vi "Data2Arrays.vi"(8 "error in (no error)":errorcluster, 11 "AllData":T1 {"FlukeData"."DataAnalysisArray"."TimeStamp" format="%^<%.3X\n%x>T"; "FlukeData"."ModelDataArray"."FREQUENCY" format="%#_6f"; "FlukeData"."ModelDataArray"."TimeStamp" format="%^<%.3X\n%x>T"; "FlukeData"."PMUDataArray"."FREQUENCY" format="%#_6f"; "FlukeData"."PMUDataArray"."TimeStamp" format="%^<%.3X\n%x>T"; "NISTData"."DataAnlysisArray"."Time" format="%.6f"; "NISTData"."DataAnlysisArray"."TimeStamp" format="%^<%.3X\n%x>T"; "NISTData"."DUTDataArray"."TimeStamp" format="%^<%.3X\n%x>T"; "NISTData"."DUTDataArray"."Time" format="%.6f"; "NISTData"."NIDataArray"."TimeStamp" format="%^<%.3X\n%x>T"; "NISTData"."NIDataArray"."Time" format="%.6f"}) -> (0 "error out":errorcluster, 2 "Fluke":dbl[][](array[numeric]), 3 "NIST":dbl[][](array[numeric]))   [LabVIEW 2014]
uses:
  typedefs/Alldata.ctl
  typedefs/NISTData.ctl
  typedefs/NIDataArray.ctl
  typedefs/NIData.ctl
  typedefs/PhasorRectangular.ctl
  typedefs/DUTData.ctl
  typedefs/NICalcAnalysis.ctl
  typedefs/CalcPhasorError.ctl
  typedefs/PlotDataArrays.ctl
  typedefs/PmuRawDataCluster.ctl
  typedefs/CalcAnalysis.ctl
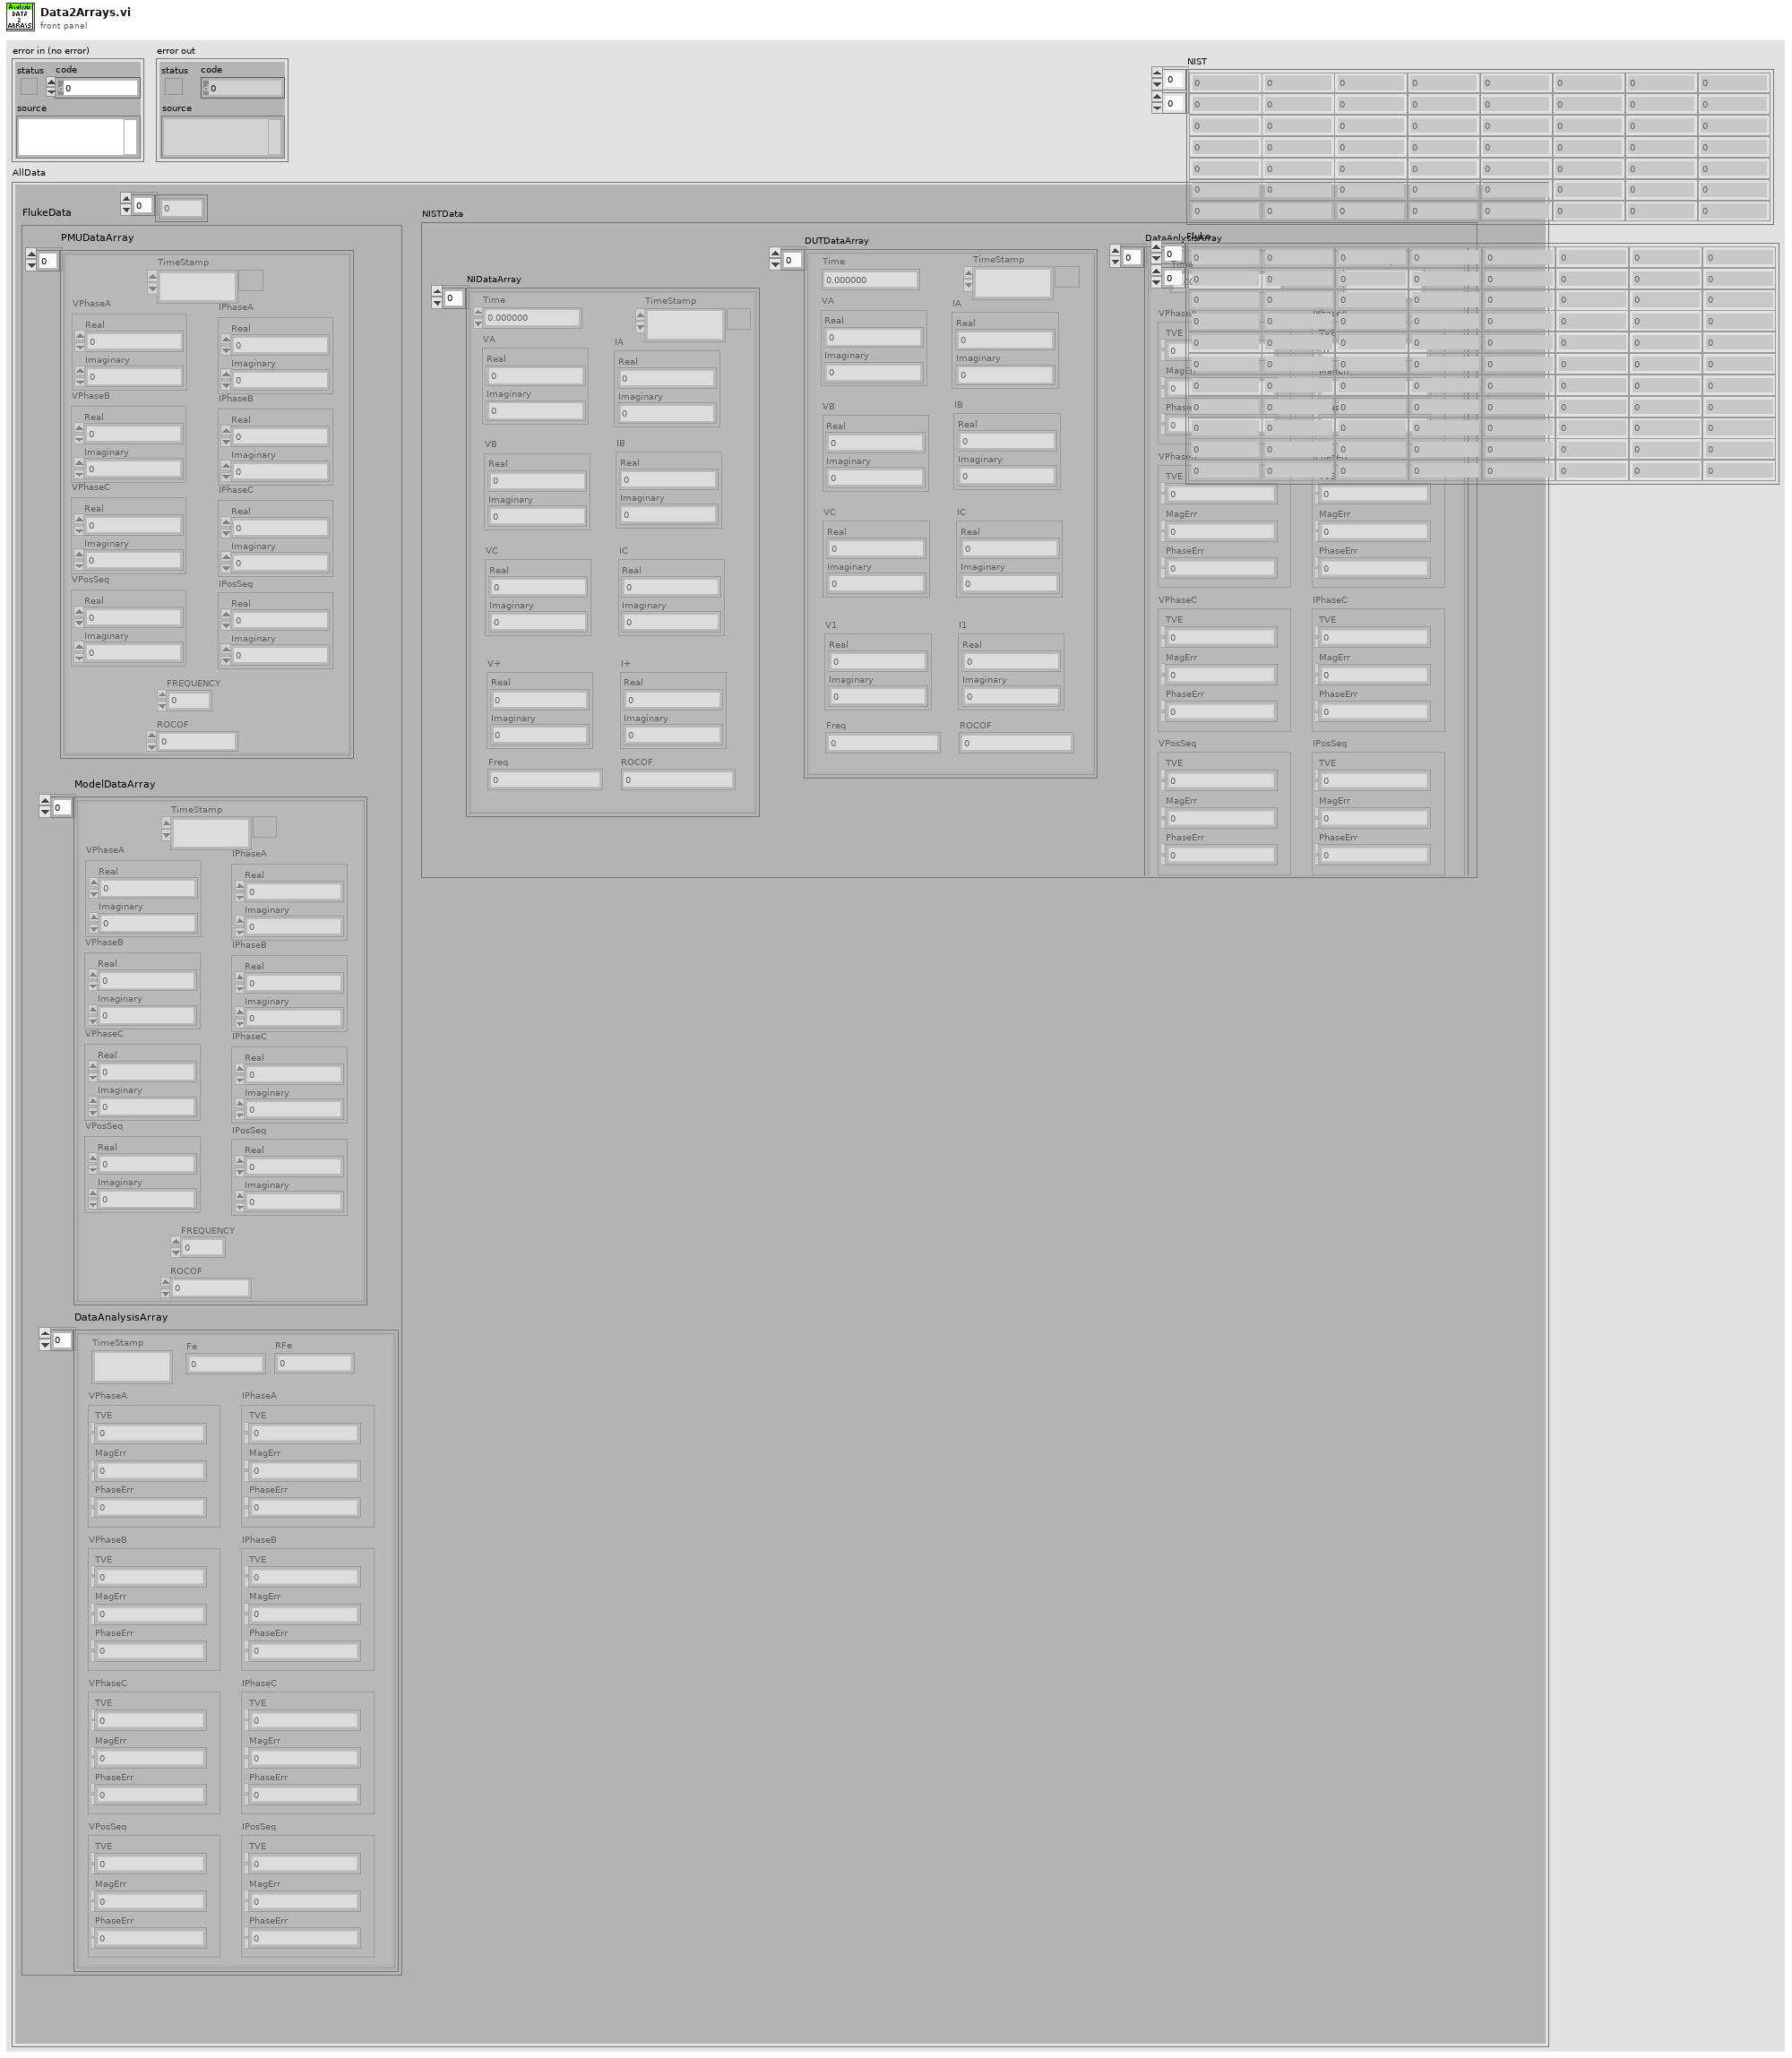
[diagram p1: front panel]
types:
  T1 = typedef "Alldata.ctl" = cluster{"NISTData":T2, "FlukeData":T9, "Params":dbl[]}
  T2 = typedef "NISTData.ctl" = cluster{"NIDataArray":T3, "DUTDataArray":T6[], "DataAnlysisArray":T7[]}
  T3 = typedef "NIDataArray.ctl" = T4[]
  T4 = typedef "NIData.ctl" = cluster{"Time":dbl, "VA":T5, "VB":T5, "VC":T5, "V+":T5, "IA":T5, "IB":T5, "IC":T5, "I+":T5, "Freq":dbl, "ROCOF":dbl, "TimeStamp":timestamp}
  T5 = typedef "PhasorRectangular.ctl" = cluster{"Real":dbl, "Imaginary":dbl}
  T6 = typedef "DUTData.ctl" = cluster{"Time":dbl, "VA":T5, "VB":T5, "VC":T5, "V1":T5, "IA":T5, "IB":T5, "IC":T5, "I1":T5, "Freq":dbl, "ROCOF":dbl, "TimeStamp":timestamp}
  T7 = typedef "NICalcAnalysis.ctl" = cluster{"Time":dbl, "VPhaseA":T8, "VPhaseB":T8, "VPhaseC":T8, "VPosSeq":T8, "IPhaseA":T8, "IPhaseB":T8, "IPhaseC":T8, "IPosSeq":T8, "Fe":dbl, "RFe":dbl, "TimeStamp":timestamp}
  T8 = typedef "CalcPhasorError.ctl" = cluster{"TVE":dbl, "MagErr":dbl, "PhaseErr":dbl}
  T9 = typedef "PlotDataArrays.ctl" = cluster{"PMUDataArray":T10[], "ModelDataArray":T10[], "DataAnalysisArray":T11[]}
  T10 = typedef "PmuRawDataCluster.ctl" = cluster{"TimeStamp":timestamp, "VPhaseA":T5, "VPhaseB":T5, "VPhaseC":T5, "VPosSeq":T5, "IPhaseA":T5, "IPhaseB":T5, "IPhaseC":T5, "IPosSeq":T5, "FREQUENCY":dbl, "ROCOF":sgl}
  T11 = typedef "CalcAnalysis.ctl" = cluster{"TimeStamp":timestamp, "VPhaseA":T8, "VPhaseB":T8, "VPhaseC":T8, "VPosSeq":T8, "IPhaseA":T8, "IPhaseB":T8, "IPhaseC":T8, "IPosSeq":T8, "Fe":dbl, "RFe":dbl}
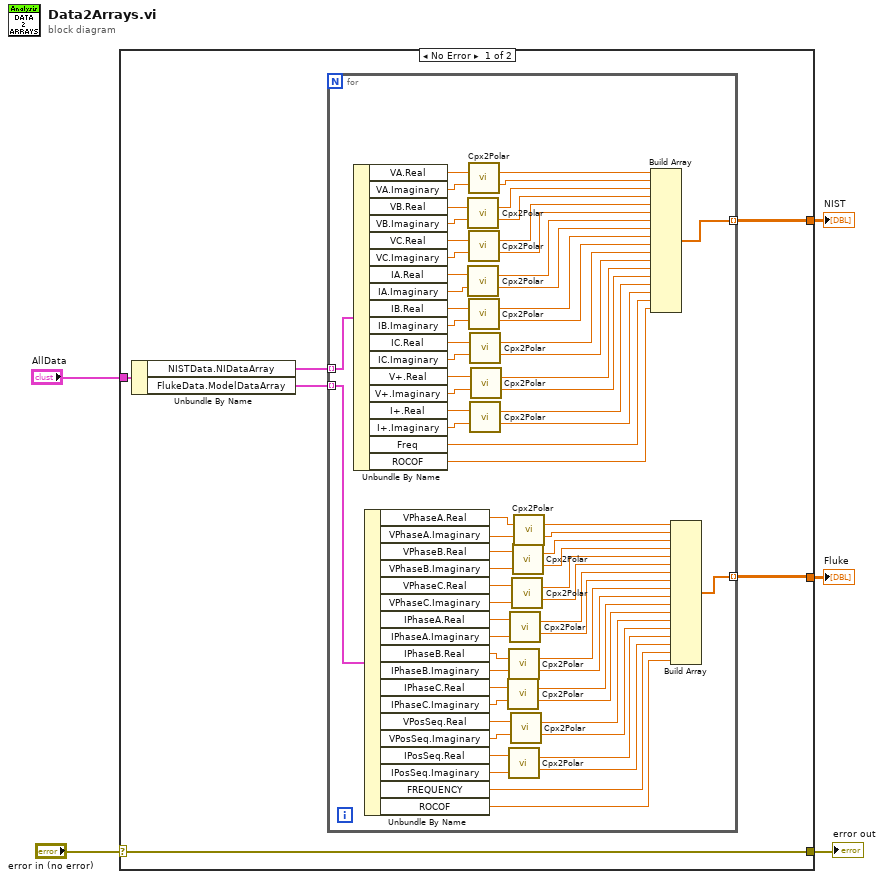
[diagram p0: block diagram]
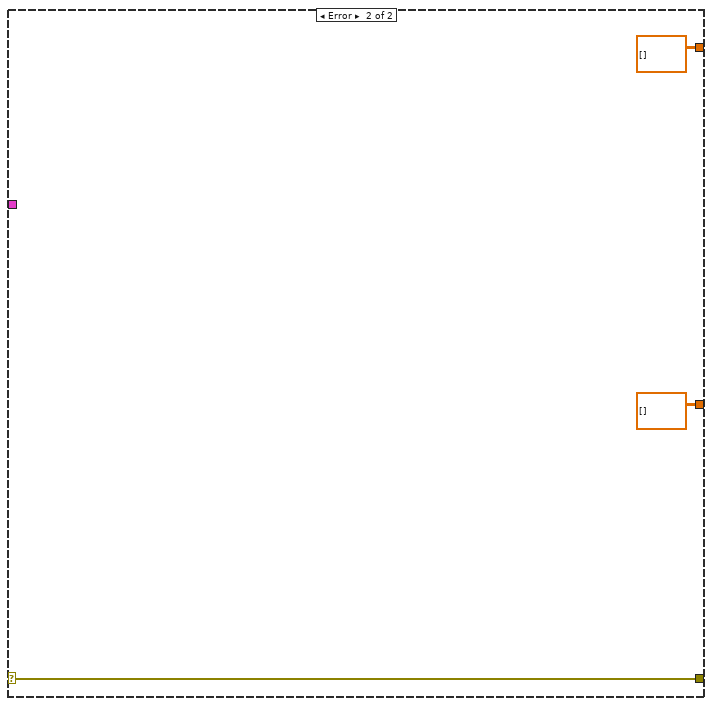
[diagram p2: hidden frame]
diagram:
  n1 = case shown="No Error" "error in (no error)" {
    selector: "error in (no error)" -> [w6 w86]
    tunnel: [w6 w86] -> w4
    tunnel: "AllData" -> [w11 _]
    tunnel: [w8 dbl[][] []] -> w2
    tunnel: [w7 dbl[][] []] -> w1
    frame No Error {
      n2 = Unbundle By Name(w11) -> ("NISTData.NIDataArray"=w10:T3, "FlukeData.ModelDataArray"=w9:T10[])
      n3 = for {
        tunnel: w10 -> [w83] mode=indexing
        tunnel: w9 -> [w82] mode=indexing
        tunnel: [w69] -> w8 mode=indexing
        tunnel: [w56] -> w7 mode=indexing
        n4 = Unbundle By Name(w83) -> ("VA.Real"=w55:dbl, "VA.Imaginary"=w54:dbl, "VB.Real"=w53:dbl, "VB.Imaginary"=w52:dbl, "VC.Real"=w51:dbl, "VC.Imaginary"=w49:dbl, "IA.Real"=w50:dbl, "IA.Imaginary"=w48:dbl, "IB.Real"=w47:dbl, "IB.Imaginary"=w46:dbl, "IC.Real"=w45:dbl, "IC.Imaginary"=w44:dbl, "V+.Real"=w21:dbl, "V+.Imaginary"=w20:dbl, "I+.Real"=w19:dbl, "I+.Imaginary"=w18:dbl, "Freq"=w13:dbl, "ROCOF"=w12:dbl)
        n5 = Unbundle By Name(w82) -> ("VPhaseA.Real"=w81:dbl, "VPhaseA.Imaginary"=w80:dbl, "VPhaseB.Real"=w79:dbl, "VPhaseB.Imaginary"=w78:dbl, "VPhaseC.Real"=w77:dbl, "VPhaseC.Imaginary"=w76:dbl, "IPhaseA.Real"=w75:dbl, "IPhaseA.Imaginary"=w74:dbl, "IPhaseB.Real"=w73:dbl, "IPhaseB.Imaginary"=w72:dbl, "IPhaseC.Real"=w71:dbl, "IPhaseC.Imaginary"=w70:dbl, "VPosSeq.Real"=w31:dbl, "VPosSeq.Imaginary"=w30:dbl, "IPosSeq.Real"=w29:dbl, "IPosSeq.Imaginary"=w28:dbl, "FREQUENCY"=w23:dbl, "ROCOF"=w22:sgl)
        n6 = call "Cpx2Polar.vi"("Real"=w53, "Imag"=w52) -> ("Mag"=w41:dbl, "Phase"=w40:dbl)  [unwired: 12 in]
        n7 = call "Cpx2Polar.vi"("Real"=w50, "Imag"=w48) -> ("Mag"=w37:dbl, "Phase"=w36:dbl)  [unwired: 12 in]
        n8 = call "Cpx2Polar.vi"("Real"=w55, "Imag"=w54) -> ("Mag"=w43:dbl, "Phase"=w42:dbl)  [unwired: 12 in]
        n9 = call "Cpx2Polar.vi"("Real"=w51, "Imag"=w49) -> ("Mag"=w39:dbl, "Phase"=w38:dbl)  [unwired: 12 in]
        n10 = call "Cpx2Polar.vi"("Real"=w47, "Imag"=w46) -> ("Mag"=w35:dbl, "Phase"=w34:dbl)  [unwired: 12 in]
        n11 = call "Cpx2Polar.vi"("Real"=w45, "Imag"=w44) -> ("Mag"=w33:dbl, "Phase"=w32:dbl)  [unwired: 12 in]
        n12 = call "Cpx2Polar.vi"("Real"=w19, "Imag"=w18) -> ("Mag"=w15:dbl, "Phase"=w14:dbl)  [unwired: 12 in]
        n13 = call "Cpx2Polar.vi"("Real"=w21, "Imag"=w20) -> ("Mag"=w17:dbl, "Phase"=w16:dbl)  [unwired: 12 in]
        n14 = call "Cpx2Polar.vi"("Real"=w71, "Imag"=w70) -> ("Mag"=w58:dbl, "Phase"=w57:dbl)  [unwired: 12 in]
        n15 = call "Cpx2Polar.vi"("Real"=w73, "Imag"=w72) -> ("Mag"=w60:dbl, "Phase"=w59:dbl)  [unwired: 12 in]
        n16 = call "Cpx2Polar.vi"("Real"=w29, "Imag"=w28) -> ("Mag"=w25:dbl, "Phase"=w24:dbl)  [unwired: 12 in]
        n17 = call "Cpx2Polar.vi"("Real"=w75, "Imag"=w74) -> ("Mag"=w62:dbl, "Phase"=w61:dbl)  [unwired: 12 in]
        n18 = call "Cpx2Polar.vi"("Real"=w31, "Imag"=w30) -> ("Mag"=w27:dbl, "Phase"=w26:dbl)  [unwired: 12 in]
        n19 = call "Cpx2Polar.vi"("Real"=w77, "Imag"=w76) -> ("Mag"=w64:dbl, "Phase"=w63:dbl)  [unwired: 12 in]
        n20 = call "Cpx2Polar.vi"("Real"=w79, "Imag"=w78) -> ("Mag"=w66:dbl, "Phase"=w65:dbl)  [unwired: 12 in]
        n21 = call "Cpx2Polar.vi"("Real"=w81, "Imag"=w80) -> ("Mag"=w68:dbl, "Phase"=w67:dbl)  [unwired: 12 in]
        n22 = Build Array(w43, w42, w41, w40, w39, w38, w37, w36, w35, w34, w33, w32, w17, w16, w15, w14, w13, w12) -> (w69:dbl[])
        n23 = Build Array(w68, w67, w66, w65, w64, w63, w62, w61, w60, w59, w58, w57, w27, w26, w25, w24, w23, w22) -> (w56:dbl[])
      }
    }
    frame Error {
    }
  }
  "error out" <- w4
  "NIST" <- w2
  "Fluke" <- w1
